vi "Servo 3.vi"(8 "error in (no error)":errorcluster, 10 "Servo":T1 {"Servo 3" min=0.0 max=255.0 step=1.0; "Servo 2" min=0.0 max=255.0 step=1.0; "Servo 1" min=0.0 max=255.0 step=1.0}, 11 "PWM in":T3) -> (0 "error out":errorcluster, 3 "PWM out":T2)   [LabVIEW 2020]
uses:
  <vilib>/High Genius/HG_WSI_Tookit/Dependencies/Library/PWM/PWM.lvclass
  C:/Program Files (x86)/National Instruments/LabVIEW 2020/vi.lib/High Genius/HG_WSI_Tookit/Dependencies/Library/HG_LIB/HG_LIB.lvclass
  <vilib>/High Genius/HG_WSI_Tookit/Dependencies/Library/HG_LIB/HG_LIB.lvclass/HG_LIB.ctl
  <vilib>/High Genius/HG_WSI_Tookit/Dependencies/Library/HG_LIB/HG_LIB.lvclass
  <vilib>/High Genius/HG_WSI_Tookit/Dependencies/Library/VMX Library.lvlib
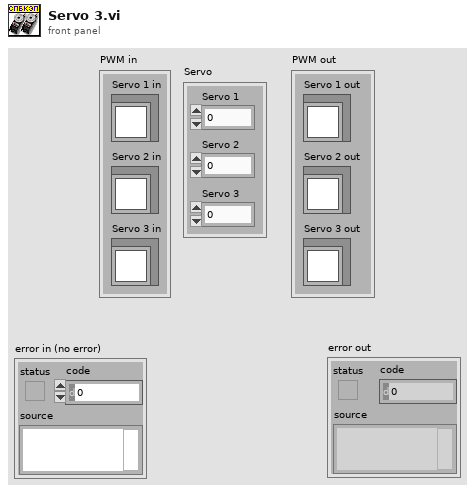
[diagram p1: front panel]
types:
  T1 = cluster{"Servo 1":dbl, "Servo 2":dbl, "Servo 3":dbl}
  T2 = cluster{"Servo 1 out":refnum<class "PWM.lvclass">, "Servo 2 out":refnum<class "PWM.lvclass">, "Servo 3 out":refnum<class "PWM.lvclass">}
  T3 = cluster{"Servo 1 in":refnum<class "PWM.lvclass">, "Servo 2 in":refnum<class "PWM.lvclass">, "Servo 3 in":refnum<class "PWM.lvclass">}
  T4 = typedef "Semaphore RefNum" = refnum<k1>
  T5 = cluster{"titanenc0":i32, "titanenc1":i32, "titanenc2":i32, "titanenc3":i32, "rpm0":i16, "rpm1":i16, "rpm2":i16, "rpm3":i16, "resetenc0":bool, "resetenc1":bool, "resetenc2":bool, "resetenc3":bool}
  T6 = cluster{"data":cluster{"ai22":sgl, "ai23":sgl, "ai24":sgl, "ai25":sgl, "pulse12":i32, "pulse13":i32, "pwm14":i32, "pwm15":i32, "pwm16":dbl, "do17":bool, "do18":bool, "do19":bool, "do20":bool, "do21":bool, "di11":bool, "di9":bool, "motor0":u8, "motor1":u8, "motor2":u8, "motor3":u8, "dir00":u8, "dir01":u8, "dir02":u8, "dir03":u8, "dir10":u8, "dir11":u8, "dir12":u8, "dir13":u8, "limit0":bool, "limit1":bool, "limit2":bool, "limit3":bool, "limit4":bool, "limit5":bool, "limit6":bool, "limit7":bool, "lsb0H":u8, "lsb1H":u8, "lsb2H":u8, "lsb3H":u8, "lsb0L":u8, "lsb1L":u8, "lsb2L":u8, "lsb3L":u8, "enc0_counters":u32, "enc1_counters":u32, "enc2_counters":u32, "enc3_counters":u32, "counter10":u32, "counter8":u32, "reset_enc0":bool, "reset_enc1":bool, "reset_enc2":bool, "reset_enc3":bool, "pitch":sgl, "roll":sgl, "yaw":sgl, "zero_yaw":bool}}
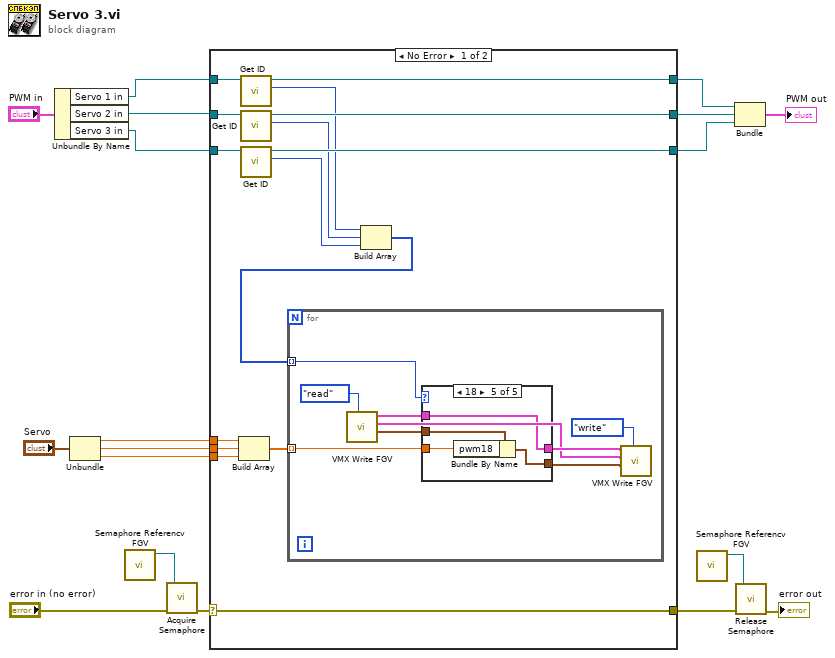
[diagram p0: block diagram]
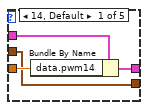
[diagram p2: hidden frame]
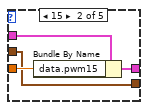
[diagram p3: hidden frame]
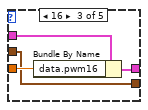
[diagram p4: hidden frame]
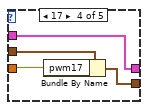
[diagram p5: hidden frame]
diagram:
  n1 = Unbundle By Name("PWM in") -> ("Servo 1 in"=w3:refnum<class "PWM.lvclass">, "Servo 2 in"=w2:refnum<class "PWM.lvclass">, "Servo 3 in"=w1:refnum<class "PWM.lvclass">)
  n2 = Unbundle("Servo") -> ("Servo 1"=w7:dbl, "Servo 2"=w6:dbl, "Servo 3"=w5:dbl)
  n3 = call <vilib>:"Semaphore Referencv FGV.vi"() -> ("Semaphore Reference"=w16:T4)  [unwired: 11 in]
  n4 = call <vilib>:"Acquire Semaphore.vi"("error in (no error)"="error in (no error)", "semaphore"=w16) -> ("error out"=w18:errorcluster)  [unwired: 3 in, 2 out]
  n5 = case shown="No Error" w18 {
    selector: w18 -> [w33 w66]
    tunnel: [w33 w66] -> w14
    tunnel: w3 -> [w32 w65]
    tunnel: [w31 w65] -> w11
    tunnel: w2 -> [w30 w64]
    tunnel: w1 -> [w29 w63]
    tunnel: [w28 w64] -> w10
    tunnel: [w27 w63] -> w9
    tunnel: w7 -> [w22 _]
    tunnel: w6 -> [w21 _]
    tunnel: w5 -> [w20 _]
    frame No Error {
      n6 = Build Array(w22, w21, w20) -> (w19:dbl[])
      n7 = call <vilib>:"Get ID.vi"("HG_LIB in"=w32) -> ("ID"=w26:u32, "HG_LIB out"=w31:refnum<class "PWM.lvclass">)  [unwired: 9 in]
      n8 = call <vilib>:"Get ID.vi"("HG_LIB in"=w30) -> ("ID"=w25:u32, "HG_LIB out"=w28:refnum<class "PWM.lvclass">)  [unwired: 9 in]
      n9 = call <vilib>:"Get ID.vi"("HG_LIB in"=w29) -> ("ID"=w24:u32, "HG_LIB out"=w27:refnum<class "PWM.lvclass">)  [unwired: 9 in]
      n10 = Build Array(w26, w25, w24) -> (w23:u32[])
      n11 = for {
        tunnel: w23 -> [w42] mode=indexing
        tunnel: w19 -> [w41] mode=indexing
        n12 = call <vilib>:"VMX Write FGV.vi"("Enum"=enum16{"read", "write"}."read") -> ("Read Data3"=w39:cluster{"pwm17":i32, "pwm18":i32}, "Read Data2"=w36:T5, "Read Data"=w40:T6)  [unwired: 8 in]
        n13 = case shown="18" w42 {
          tunnel: [w46 w49 w51 w57 w61] -> w37
          tunnel: w41 -> [w45 w50 w54 w58 w62]
          tunnel: w40 -> [w44 w47 w53 w57 w61]
          tunnel: w39 -> [w43 w48 w52 w56 w59]
          tunnel: [w43 w48 w52 w55 w60] -> w35
          frame 14, Default {
            n14 = Bundle By Name(cluster=w44, "data.pwm14"=w45) -> (w46:T6)
          }
          frame 15 {
            n15 = Bundle By Name(cluster=w47, "data.pwm15"=w50) -> (w49:T6)
          }
          frame 16 {
            n16 = Bundle By Name(cluster=w53, "data.pwm16"=w54) -> (w51:T6)
          }
          frame 17 {
            n17 = Bundle By Name(cluster=w56, "pwm17"=w58) -> (w55:cluster{"pwm17":i32, "pwm18":i32})
          }
          frame 18 {
            n18 = Bundle By Name(cluster=w59, "pwm18"=w62) -> (w60:cluster{"pwm17":i32, "pwm18":i32})
          }
        }
        n19 = call <vilib>:"VMX Write FGV.vi"("Enum"=enum16{"read", "write"}."write", "Write Data3"=w35, "Write Data2"=w36, "Write Data"=w37) -> ()  [unwired: 5 in, 3 out]
      }
    }
    frame Error {
    }
  }
  n20 = call <vilib>:"Semaphore Referencv FGV.vi"() -> ("Semaphore Reference"=w15:T4)  [unwired: 11 in]
  n21 = Bundle("Servo 1 in"=w11, "Servo 2 in"=w10, "Servo 3 in"=w9) -> (→"PWM out":T3)  [unwired: 1 in]
  n22 = call <vilib>:"Release Semaphore.vi"("error in (no error)"=w14, "semaphore"=w15) -> ("error out"=→"error out":errorcluster)  [unwired: 4 in, 1 out]
